vi "Get Size with Offset.vi"(8 "error in (no error)":errorcluster, 11 "Channel Configuration in":refnum<class "Configuration.Channel.lvclass">) -> (0 "error out":errorcluster, 2 "size+offset in bytes":u64, 3 "Channel Configuration out":refnum<class "Configuration.Channel.lvclass">)   [LabVIEW 2016, in "Configuration.Channel.lvclass"]
uses:
  Configuration.Channel.lvclass
  Configuration.Channel.lvclass/Configuration.Channel.ctl
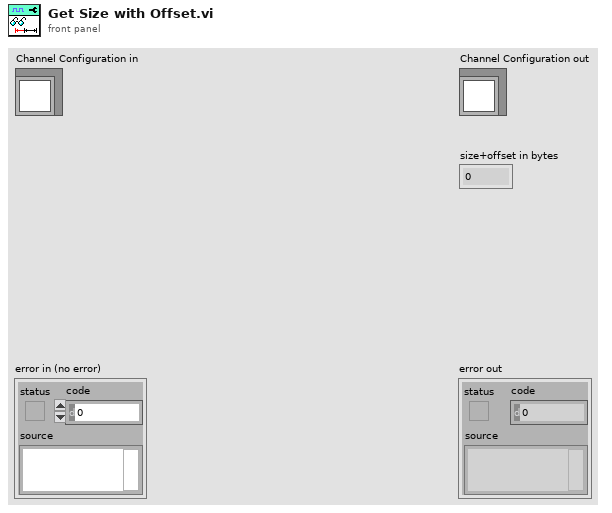
[diagram p1: front panel]
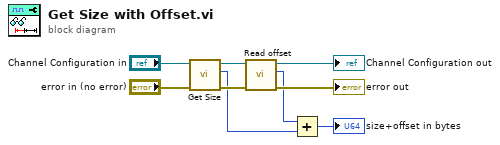
[diagram p0: block diagram]
diagram:
  n1 = call "Get Size.vi"("error in (no error)"="error in (no error)", "Channel Configuration in"="Channel Configuration in") -> ("error out"=w6:errorcluster, "size in bytes"=w2:u64, "Channel Configuration out"=w7:refnum<class "Configuration.Channel.lvclass">)  [unwired: 7 in]
  n2 = call "Read offset.vi"("error in (no error)"=w6, "Configuration.Channel in"=w7) -> ("error out"=→"error out":errorcluster, "offset"=w3:u64, "Configuration.Channel out"=→"Channel Configuration out":refnum<class "Configuration.Channel.lvclass">)  [unwired: 7 in]
  n3 = Add(x=w3, y=w2) -> (x+y=→"size+offset in bytes":u64)
